vi "ErrorMessageBuilder.vi"(1 "Errors":T1(array[cluster])) -> (0 "Combined Error String":string)   [LabVIEW 2019]
doc: "This VI is used to convert a set of boolean triggers into an error message string which may be displayed or spoken aloud. The error messages will repeat with a period set by \"Delays.\""
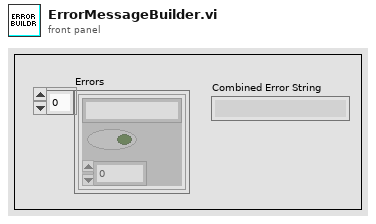
[diagram p1: front panel]
types:
  T1 = cluster{"Error Message":string, "Trigger":bool, "Delay (s)":dbl}[]
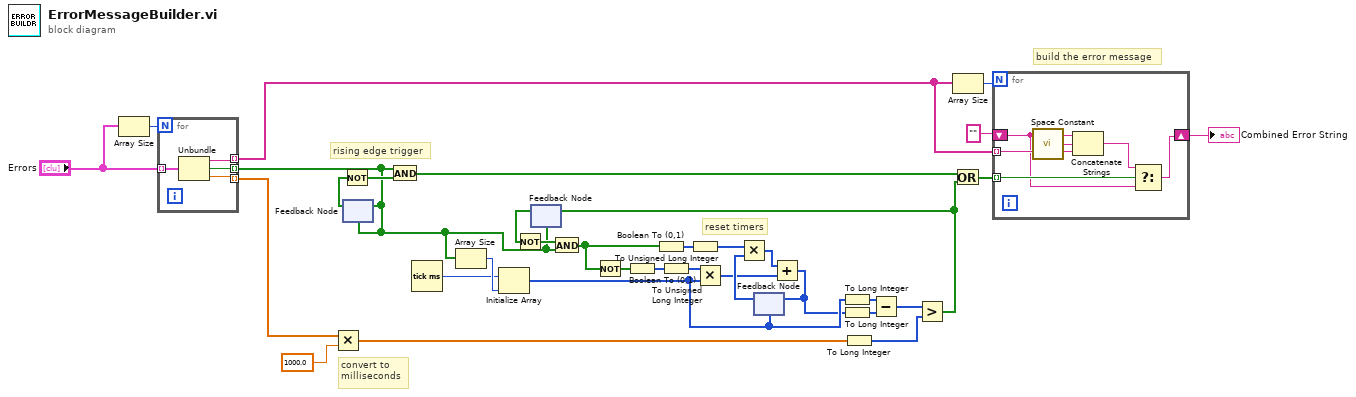
[diagram p0: block diagram]
diagram:
  # "convert to\nmilliseconds"
  # "build the error message"
  # "reset timers"
  # "rising edge trigger"
  n1 = Array Size(array="Errors") -> (size(s)=w5:i32)
  n2 = for {
    N: w5 -> [_]
    tunnel: "Errors" -> [w38] mode=indexing
    tunnel: [w37] -> w3 mode=indexing
    tunnel: [w36] -> w2 mode=indexing
    tunnel: [w35] -> w1 mode=indexing
    n3 = Unbundle(w38) -> ("Error Message"=w36:string, "Trigger"=w37:bool, "Delay (s)"=w35:dbl)
  }
  n4 = Multiply(x=w1, y=1000.0) -> (x*y=w7:dbl[])
  n5 = feedback #1(w3) -> (w9:bool[])
  n6 = Not(x=w9) -> (.not. x?=w27:bool[])
  n7 = feedback-in #1(w3) -> ()
  n8 = And(x=w3, y=w27) -> (x .and. y?=w33:bool[])
  n9 = Tick Count (ms)() -> (millisecond timer value=w12:u32)
  n10 = Array Size(array=w3) -> (size(s)=w25:i32)
  n11 = Initialize Array(w12, w25) -> (w23:u32[])
  n12 = feedback #2(w3) -> (w30:bool[])
  n13 = Not(x=w30) -> (.not. x?=w31:bool[])
  n14 = And(x=w31, y=w3) -> (x .and. y?=w29:bool[])
  n15 = Not(x=w29) -> (.not. x?=w28:bool[])
  n16 = Boolean To (0,1)(Boolean=w28) -> (0, 1=w13:i16[])
  n17 = Boolean To (0,1)(Boolean=w29) -> (0, 1=w15:i16[])
  n18 = To Unsigned Long Integer(number=w13) -> (unsigned 32bit integer=w14:u32[])
  n19 = To Unsigned Long Integer(number=w15) -> (unsigned 32bit integer=w17:u32[])
  n20 = Multiply(x=w14, y=w23) -> (x*y=w16:u32[])
  n21 = feedback #3(w23) -> (w18:u32[])
  n22 = Multiply(x=w17, y=w18) -> (x*y=w19:u32[])
  n23 = Add(x=w19, y=w16) -> (x+y=w22:u32[])
  n24 = feedback-in #3(w22) -> ()
  n25 = To Long Integer(number=w23) -> (32bit integer=w20:i32[])
  n26 = To Long Integer(number=w22) -> (32bit integer=w21:i32[])
  n27 = To Long Integer(number=w7) -> (32bit integer=w26:i32[])
  n28 = Subtract(x=w20, y=w21) -> (x-y=w24:i32[])
  n29 = Greater?(x=w24, y=w26) -> (0:w32:bool[])
  n30 = feedback-in #2(w32) -> ()
  n31 = Array Size(array=w2) -> (size(s)=w8:i32)
  n32 = Or(x=w33, y=w32) -> (x .or. y?=w34:bool[])
  n33 = for {
    N: w8 -> [_]
    tunnel: w34 -> [w44] mode=indexing
    tunnel: w2 -> [w42] mode=indexing
    shift-right: [w40] -> w10
    shift-left: "" -> [w39]
    n34 = call <vilib>:"Space Constant.vi"() -> ("String"=w43:string)
    n35 = Concatenate Strings(w39, w43, w42) -> (w41:string)
    n36 = Select(t=w41, s=w44, f=w39) -> (s? t:f=w40:string)
  }
  "Combined Error String" <- w10
